vi "Set Pulse Width.vi"(8 "error in (no error)":errorcluster, 10 "pulse width (micro-sec)":dbl, 11 "Servo in":refnum<class "Servo.lvclass">) -> (0 "error out":errorcluster, 3 "Servo out":refnum<class "Servo.lvclass">)   [LabVIEW 2020, in "Servo.lvclass"]
uses:
  Servo.lvclass
  Servo.lvclass/Servo.ctl
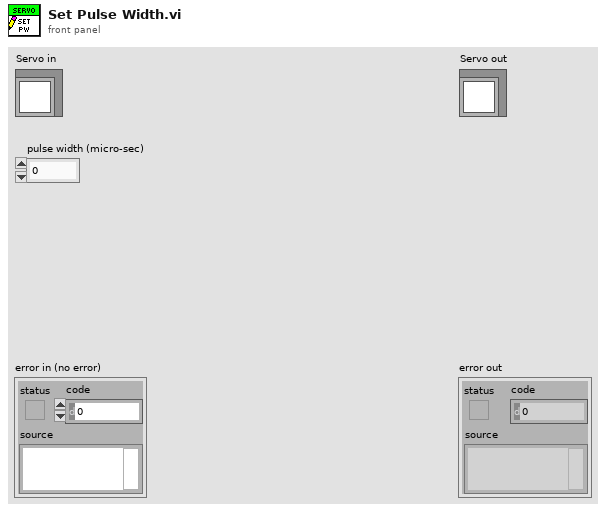
[diagram p1: front panel]
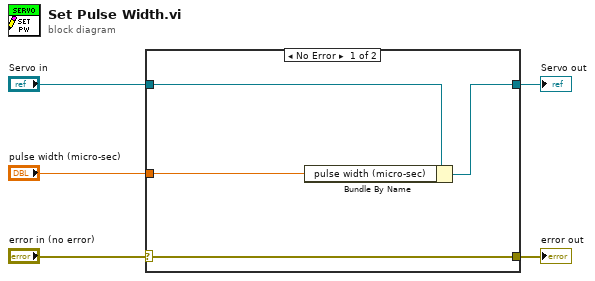
[diagram p0: block diagram]
diagram:
  n1 = case shown="No Error" "error in (no error)" {
    selector: "error in (no error)" -> [w9 w10]
    tunnel: [w9 w10] -> w4
    tunnel: [w7 w11] -> w2
    tunnel: "Servo in" -> [w8 w11]
    tunnel: "pulse width (micro-sec)" -> [w6 _]
    frame No Error {
      n2 = Bundle By Name(cluster=w8, "pulse width (micro-sec)"=w6) -> (w7:refnum<class "Servo.lvclass">)
    }
    frame Error {
    }
  }
  "error out" <- w4
  "Servo out" <- w2
